vi "Robust linear fit.vi"() -> ()   [LabVIEW 2014]
doc: "This example shows the effect of a single outlier on a linear fit."
uses:
  <vilib>/Analysis/1siggen.llb/Ramp Pattern by Samples.vi
  <vilib>/Analysis/NI_AALPro.lvlib
  <vilib>/Analysis/NI_AALBase.lvlib
panel:
  out "XY Graph":T1(graph)
  in  "Stop":bool
  out "fit intercept":dbl format="%#.6g"
  out "fit slope":dbl format="%#.6g"
  in  "Method":u16(ring) items=["Least Square", "Least Absolute Residual", "Bisquare"]
  in  "Add Outlier?":bool
  in  "intercept":dbl=1.0
  in  "slope":dbl=0.23
  # "Overview: This example shows the effect of a single outlier on a linear fit, and how to overcome the disproportionate effect of the outlier on the fit.  \nRequirements: LabVIEW Full Development System\nInstructions:\n1. Run the VI.\n2. Change the Method value to 'Least Absolute Residual', then 'Bisquare'. Observe that the different methods give the same result.\n3. Change the Method value to 'Least Square', and click Add Outlier?. Observe the poor quality of the fit.\n4. Change the Method value to 'Least Absolute Residual', then 'Bisquare'. Observe the improved fit.\n5. Click Stop to stop the VI."
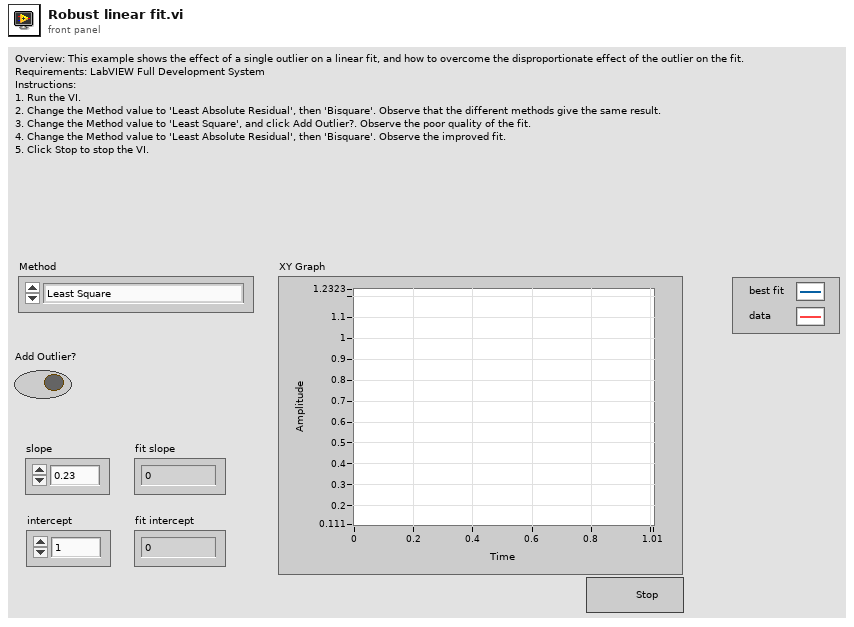
[diagram p1: front panel]
types:
  T1 = cluster{"Ramp Pattern":dbl[], "Best Linear Fit":dbl[]}[]
  T2 = cluster{"Ramp Pattern":dbl[], "Best Linear Fit":dbl[]}
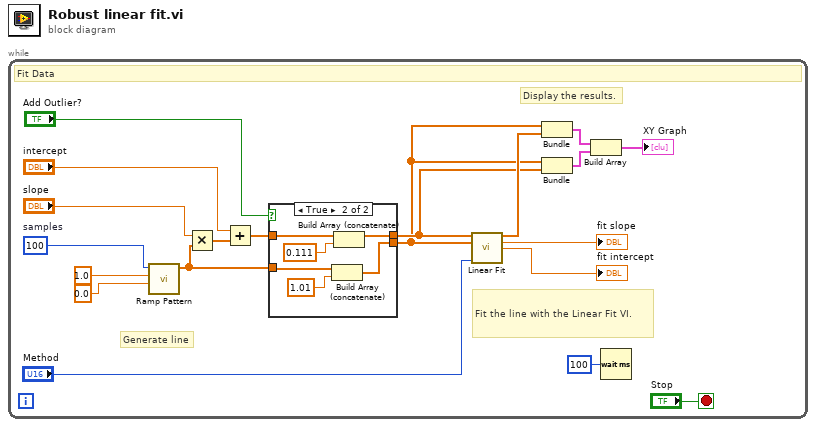
[diagram p0: block diagram]
diagram:
  n1 = while {
    stop <- "Stop" stop-if-true
    w18 = 100  # samples
    # "Display the results."
    # "Fit the line with the Linear Fit VI."
    # "Generate line"
    # "Fit Data"
    n2 = call-poly <vilib>:"Ramp Pattern.vi"("start"=0.0, "end"=1.0, "samples"=w18) -> ("Ramp Pattern"=w4:dbl[])  [unwired: 7 in, 1 out]
    n3 = Multiply(x="slope", y=w4) -> (x*y=w16:dbl[])
    n4 = Add(x="intercept", y=w16) -> (x+y=w6:dbl[])
    n5 = case shown="True" "Add Outlier?" {
      tunnel: w6 -> [w22 w28]
      tunnel: [w22 w24] -> w5
      tunnel: w4 -> [w21 w26]
      tunnel: [w21 w27] -> w3
      frame False {
      }
      frame True {
        n6 = Build Array (concatenate)(w26, 1.01) -> (w27:dbl[])
        n7 = Build Array (concatenate)(w28, 0.111) -> (w24:dbl[])
      }
    }
    n8 = call <vilib>:"Linear Fit.vi"("Y"=w5, "X"=w3, "method"="Method") -> ("Best Linear Fit"=w11:dbl[], "slope"=→"fit slope":dbl, "intercept"=→"fit intercept":dbl)  [unwired: 8 in, 2 out]
    n9 = Bundle("Ramp Pattern"=w3, "Best Linear Fit"=w11) -> (w10:T2)  [unwired: 1 in]
    n10 = Bundle("Ramp Pattern"=w3, w5) -> (w9:cluster{"Ramp Pattern":dbl[], dbl[]})  [unwired: 1 in]
    n11 = Build Array(w10, w9) -> (→"XY Graph":T1)
    n12 = Wait (ms)(milliseconds to wait=u32 100) -> ()  [unwired: 1 out]
  }
